vi "VECTOR 1610.vi"() -> ()   [LabVIEW 2020]
uses:
  SubVIs/VECTOR 1610_TypeDefinitions.llb/VECTOR 1610_XL_HWTYPE.ctl
  SubVIs/VECTOR 1610_TypeDefinitions.llb/VECTOR 1610_BitRate.ctl
  SubVIs/VECTOR 1610_TypeDefinitions.llb/VECTOR 1610_Rx_Data.ctl
  LabVIEW 2020 Toolkits/toolkits_lv2020_32bit/Synchronization.llb/SynchRefs_SetGet.ctl
  LabVIEW 2020 Toolkits/VI Server Toolkit/VI Server Libraries/VI Server_GetControl.llb/VI Server_STR_Get.vi
  LabVIEW 2020 Toolkits/VI Server Toolkit/VI Server Libraries/VI Server_Set Controls.llb/Set STR Control.vi
  LabVIEW 2020 Toolkits/VI Server Toolkit/VI Server Libraries/VI Server_GetControl.llb/VI Server_1D_Array_U8_Get.vi
  LabVIEW 2020 Toolkits/VI Server Toolkit/VI Server Libraries/VI Server_SetControl.llb/VI Server_U8_Set.vi
  LabVIEW 2020 Toolkits/VI Server Toolkit/VI Server Libraries/VI Server_GetControl.llb/VI Server_1D_Array_DBL_Get.vi
  LabVIEW 2020 Toolkits/VI Server Toolkit/VI Server Libraries/VI Server_GetControl.llb/VI Server_I32_Get.vi
  LabVIEW 2020 Toolkits/VI Server Toolkit/VI Server Libraries/VI Server_SetControl.llb/VI Server_DBL_Set.vi
  LabVIEW 2020 Toolkits/VI Server Toolkit/VI Server Toolkit LV2013.lvlib
panel:
  in  "LastAction.AddToSecuence":bool
  in  "Open.NIXNET.Database":bool
  in  "Manual.Open":bool caption="IDD.Open"
  in  "IDD.Open":bool
  in  "Help":bool
  in  "FP.Hide":bool caption="FrontPanel.Hide"
  out "System.Message":string caption="System Message"
  in  "EXIT":bool
  in  "Tab.Main":T1(tab)
  in  "TX.Payload.UpdateBytes":bool
  in  "Ch1.TX.Payload.Clear":bool
  in  "CH1.TX.Frames.Cluster":u16(ring) caption="Frames Cluster" items=["NIXNET_Development.CAN_Cluster", "NIXNET_Development.CAN_Demo_Box_Cluster", "NIXNET_Development.FlexRay_Cluster", "NIXNET_Development.J1939_Over_CAN"]
  out "CH1.TX.Signal.Comment":string caption="Comment"
  out "CH1.TX.Frame.PayloadLength":u32 caption="Payload Length"
  out "CH1.TX.Frame.Identifier":u32 caption="Identifier" format="%08x"
  in  "CH1.TX.Frame.Selector":u16(ring) caption="Frame Selector"
  out "CH1.TX.Signal.Unit":string caption="Unit"
  out "CH1.TX.Signal.DefaultValue":dbl caption="Default Value"
  out "CH1.TX.Signal.MinimumValue":dbl caption="Minimum Value"
  out "CH1.TX.Signal.MaximumValue":dbl caption="Maximum Value"
  out "CH1.TX.Signal.ScalingOffset":dbl caption="Scaling Offset"
  out "CH1.TX.Signal.ScalingFactor":dbl caption="Scaling Factor"
  out "CH1.TX.Signal.ByteOrder":u32(ring) caption="Byte Order" items=["Little Endian", "Big Endian"]
  out "CH1.TX.Signal.DataType":u32(ring) caption="Data Type" items=["Signed", "Unsigned", "IEEE Float"]
  out "CH1.TX.Signal.NumberOfBits":u32 caption="Number Of Bits"
  out "CH1.TX.Signal.StartBit":u32 caption="Start Bit"
  out "CH1.TX.Signal.Name":string caption="Name"
  in  "CH1.TX.Frame.Signals":u16(ring) caption="Frame Signals"
  in  "Ch1.TX.Transmit.Byte8":u8 caption="Byte 8" format="%02x"
  in  "Ch1.TX.Transmit.Byte7":u8 caption="Byte 7" format="%02x"
  in  "Ch1.TX.Transmit.Byte6":u8 caption="Byte 6" format="%02x"
  in  "Ch1.TX.Transmit.Byte5":u8 caption="Byte 5" format="%02x"
  in  "Ch1.TX.Transmit.Byte4":u8 caption="Byte 4" format="%02x"
  in  "Ch1.TX.Transmit.Byte3":u8 caption="Byte 3" format="%02x"
  in  "Ch1.TX.Transmit.Byte2":u8 caption="Byte 2" format="%02x"
  in  "Ch1.TX.Transmit.Byte1":u8 caption="Byte 1" format="%02x"
  in  "Ch1.TX.DataLength":u16 caption="Data Length" max=8
  in  "CH1.TX.FrameID":u32=2566838656 caption="Frame ID" format="%08x"
  in  "Ch1.TX.Payload":u8[](array[numeric]) caption="Payload" format="%02x"
  in  "CH1.TX.Signal.Data":dbl caption="Signal Data" min=0.0 max=10000.0 format="%0.3f "
  in  "Ch1.TX.Transmit":bool
  out "Ch2.ReceivedDataArray.IndexedValue":dbl caption="Value" format="%0.0f"
  in  "Ch2.ReceivedDataArray.Index":i32 caption="Index" max=6
  in  "Ch2.ReceivedDataArray.Precision":u8 caption="Precision" max=6
  out "Ch2.ReceivedDataArray":dbl[](array[numeric]) caption="Received Data Array"
  out "Ch2.Responce.String":string
  out "Ch1.Responce.Message.Checksum":string caption="Checksum"
  out "Ch1.Responce.Message.Load":string caption="PayloadLoad"
  out "Ch1.Responce.Message.Length":string caption="Length"
  out "Ch1.Responce.Message.ID":string caption="Message ID"
  out "Ch1.Responce.Message.Payload":u8[](array[numeric]) caption="Message Payload" format="%02x"
  out "CH1.RX.Signal.Data":dbl caption="Signal Data" min=0.0 max=8031.000000000005 format="%0.3f rpm"
  out "CH1.RX.Signal.Unit":string caption="Unit"
  out "CH1.RX.Signal.DefaultValue":dbl caption="Default Value"
  out "CH1.RX.Signal.MinimumValue":dbl caption="Minimum Value"
  out "CH1.RX.Signal.MaximumValue":dbl caption="Maximum Value"
  out "CH1.RX.Signal.ScalingOffset":dbl caption="Scaling Offset"
  out "CH1.RX.Signal.ScalingFactor":dbl caption="Scaling Factor"
  out "CH1.RX.Signal.ByteOrder":u32(ring) caption="Byte Order" items=["Little Endian", "Big Endian"]
  out "CH1.RX.Signal.DataType":u32(ring) caption="Data Type" items=["Signed", "Unsigned", "IEEE Float"]
  out "CH1.RX.Signal.NumberOfBits":u32 caption="Number Of Bits"
  out "CH1.RX.Signal.StartBit":u32 caption="Start Bit"
  in  "CH1.RX.FrameIDs":u16(ring) caption="Frame Id's"
  out "CH1.RX.Frame.PayloadLength":u32 caption="Payload Length"
  out "CH1.RX.Frame.Identifier":u32 caption="Identifier" format="%.0x"
  in  "CH1.RX.Frame.Selector":u16(ring) caption="Frame Selector"
  out "CH1.RX.Signal.Name":string caption="Name"
  in  "CH1.RX.Frame.Signals":u16(ring) caption="Frame Signals"
  out "CH1.RX.DATA":T2[](array[typedef]) caption="RX DATA" {"TimeStamp" format="%.0x"; "CH1.Received.Payload" format="%02x"; "CH1.Received.DataLength" max=8; "CH1.Received.FrameID" format="%08x"}
  out "CH1.RX.Signal.Comment":string caption="Comment"
  in  "CH1.RX.Frames.Cluster":u16(ring) caption="Frames Cluster" items=["NIXNET_Development.CAN_Cluster", "NIXNET_Development.CAN_Demo_Box_Cluster", "NIXNET_Development.FlexRay_Cluster", "NIXNET_Development.J1939_Over_CAN"]
  out "StringMode.Received Data":string
  in  "Argument.Precision":u8 caption="Precision" max=6
  in  "Argument.Value":dbl caption="Value"
  in  "Argument.Number":i32=1 caption="Number" min=1 max=100
  in  "Message.PrototypeString":string caption="Message Prototype String"
  in  "TestCase.Execute.All":bool
  in  "TestCase.Execute.Selected":bool
  out "TestCase.SAVE.Success":bool
  in  "TestCase.SAVE":bool
  in  "SequenceFile.Open":bool
  in  "SequenceFile":path caption="Secuence File"
  in  "TestCase.Execute.Step.Pause":bool
  in  "TestCase.Execute.Steps":u16(ring) caption="Test Case: Pause Before Step" items=["1", "2", "3", "4", "5", "6", "7", "8", "9", "10", "11", "12", "13", "14", "15", "16", "17", "18"]
  in  "TestCase.Execute.ABORT":bool
  in  "TestCase.Execute.Next":bool
  in  "TestCase.Execute.Pause":bool
  out "TestCase.ExecutionTime":dbl caption="Execution Time:" format="%0.3f sec"
  in  "TestCase.Execution.StepTime":u32 caption="Seq. Execution: Step Time" format="%d msec"
  in  "TestCaseConfiguration":i32[](listbox) caption="Test Case Configuration"
  in  "TestCase.StepDescription":string caption="Step Description:"
  in  "NIXNET.DatabaseEditor":path=path "C:/Program Files (x86)/National Instruments/NI-XNET/editor/XNetDbEd.exe" caption="NIXNET Database Editor"
  in  "Database.Selector":u16(ring) caption="Database Selector" items=["NIXNET_Development", "NIXNET_Development_1", "NIXNET_Development_2", "NIXNET_Development_3"]
  in  "BitRate":T3=125000 caption="Bit Rate" items=["20 KBd"=20000, "50 KBd"=50000, "62K5 Bd"=62500, "100 KBd"=100000, "125 KBd"=125000, "250 KBd"=250000, "500 KBd"=500000, "1 MBd"=1000000]
  in  "hwChannel.1":i32
  in  "hwIndex":i32
  in  "XL_HWTYPE":T4=55 items=["NONE"=0, "VIRTUAL"=1, "CANCARDX"=2, "CANCARDY"=12, "CANCARDXL"=15, "CANCASEXL"=21, "CANCASEXL_LOG_OBSOLETE"=23, "CANBOARDXL"=25, "CANBOARDXL_PXI"=27, "VN2600"=29, "VN3300"=37, "VN3600"=39, "VN7600"=41, "CANCARDXLE"=43, "VN8900"=45, "VN8950"=47, "VN2640"=53, "VN1610"=55, "VN1630"=57, "VN1640"=59, "VN8970"=61, "VN1611"=63, "VN5610"=65, "VN7570"=67, "IPCLIENT"=69]
  in  "VI.WindowsTitle":string caption="Windows Title"
  in  "UDP.Test.String2.Send":bool
  in  "UDP.Test.String2":string caption="UDP: Test String 2"
  in  "UDP.Port.BC":u16=58433 caption="UDP: Port.BC"
  in  "UDP.Port.RT":u16=58432 caption="UDP: Port.RT"
  in  "UDP.LocalPort.Write":u16=58434 caption="UDP: Local Port.Write"
  in  "UDP.IP.Address":string="234.5.6.7" caption="UDP: IP Address"
  in  "UDP.Test.String1.Send":bool
  in  "UDP.Test.String1":string caption="UDP: Test String 1"
  in  "UDP.Responce.String.Monitor":bool
  out "UDP.ExecEng.Message.String":string caption="UDP: Execution Engine Message String"
  out "error out":errorcluster
  in  "hwChannel.2":i32
  in  "error in":errorcluster
  # "13JUN2022"
  # "Channel 1 Send Data"
  # "Channel 1 Received Data"
  # "M"
  # "VESTOR 1610 SETTINGS"
  # "Multicast IP addresses must be in the 224.0.0.0 to 239.255.255.255 range."
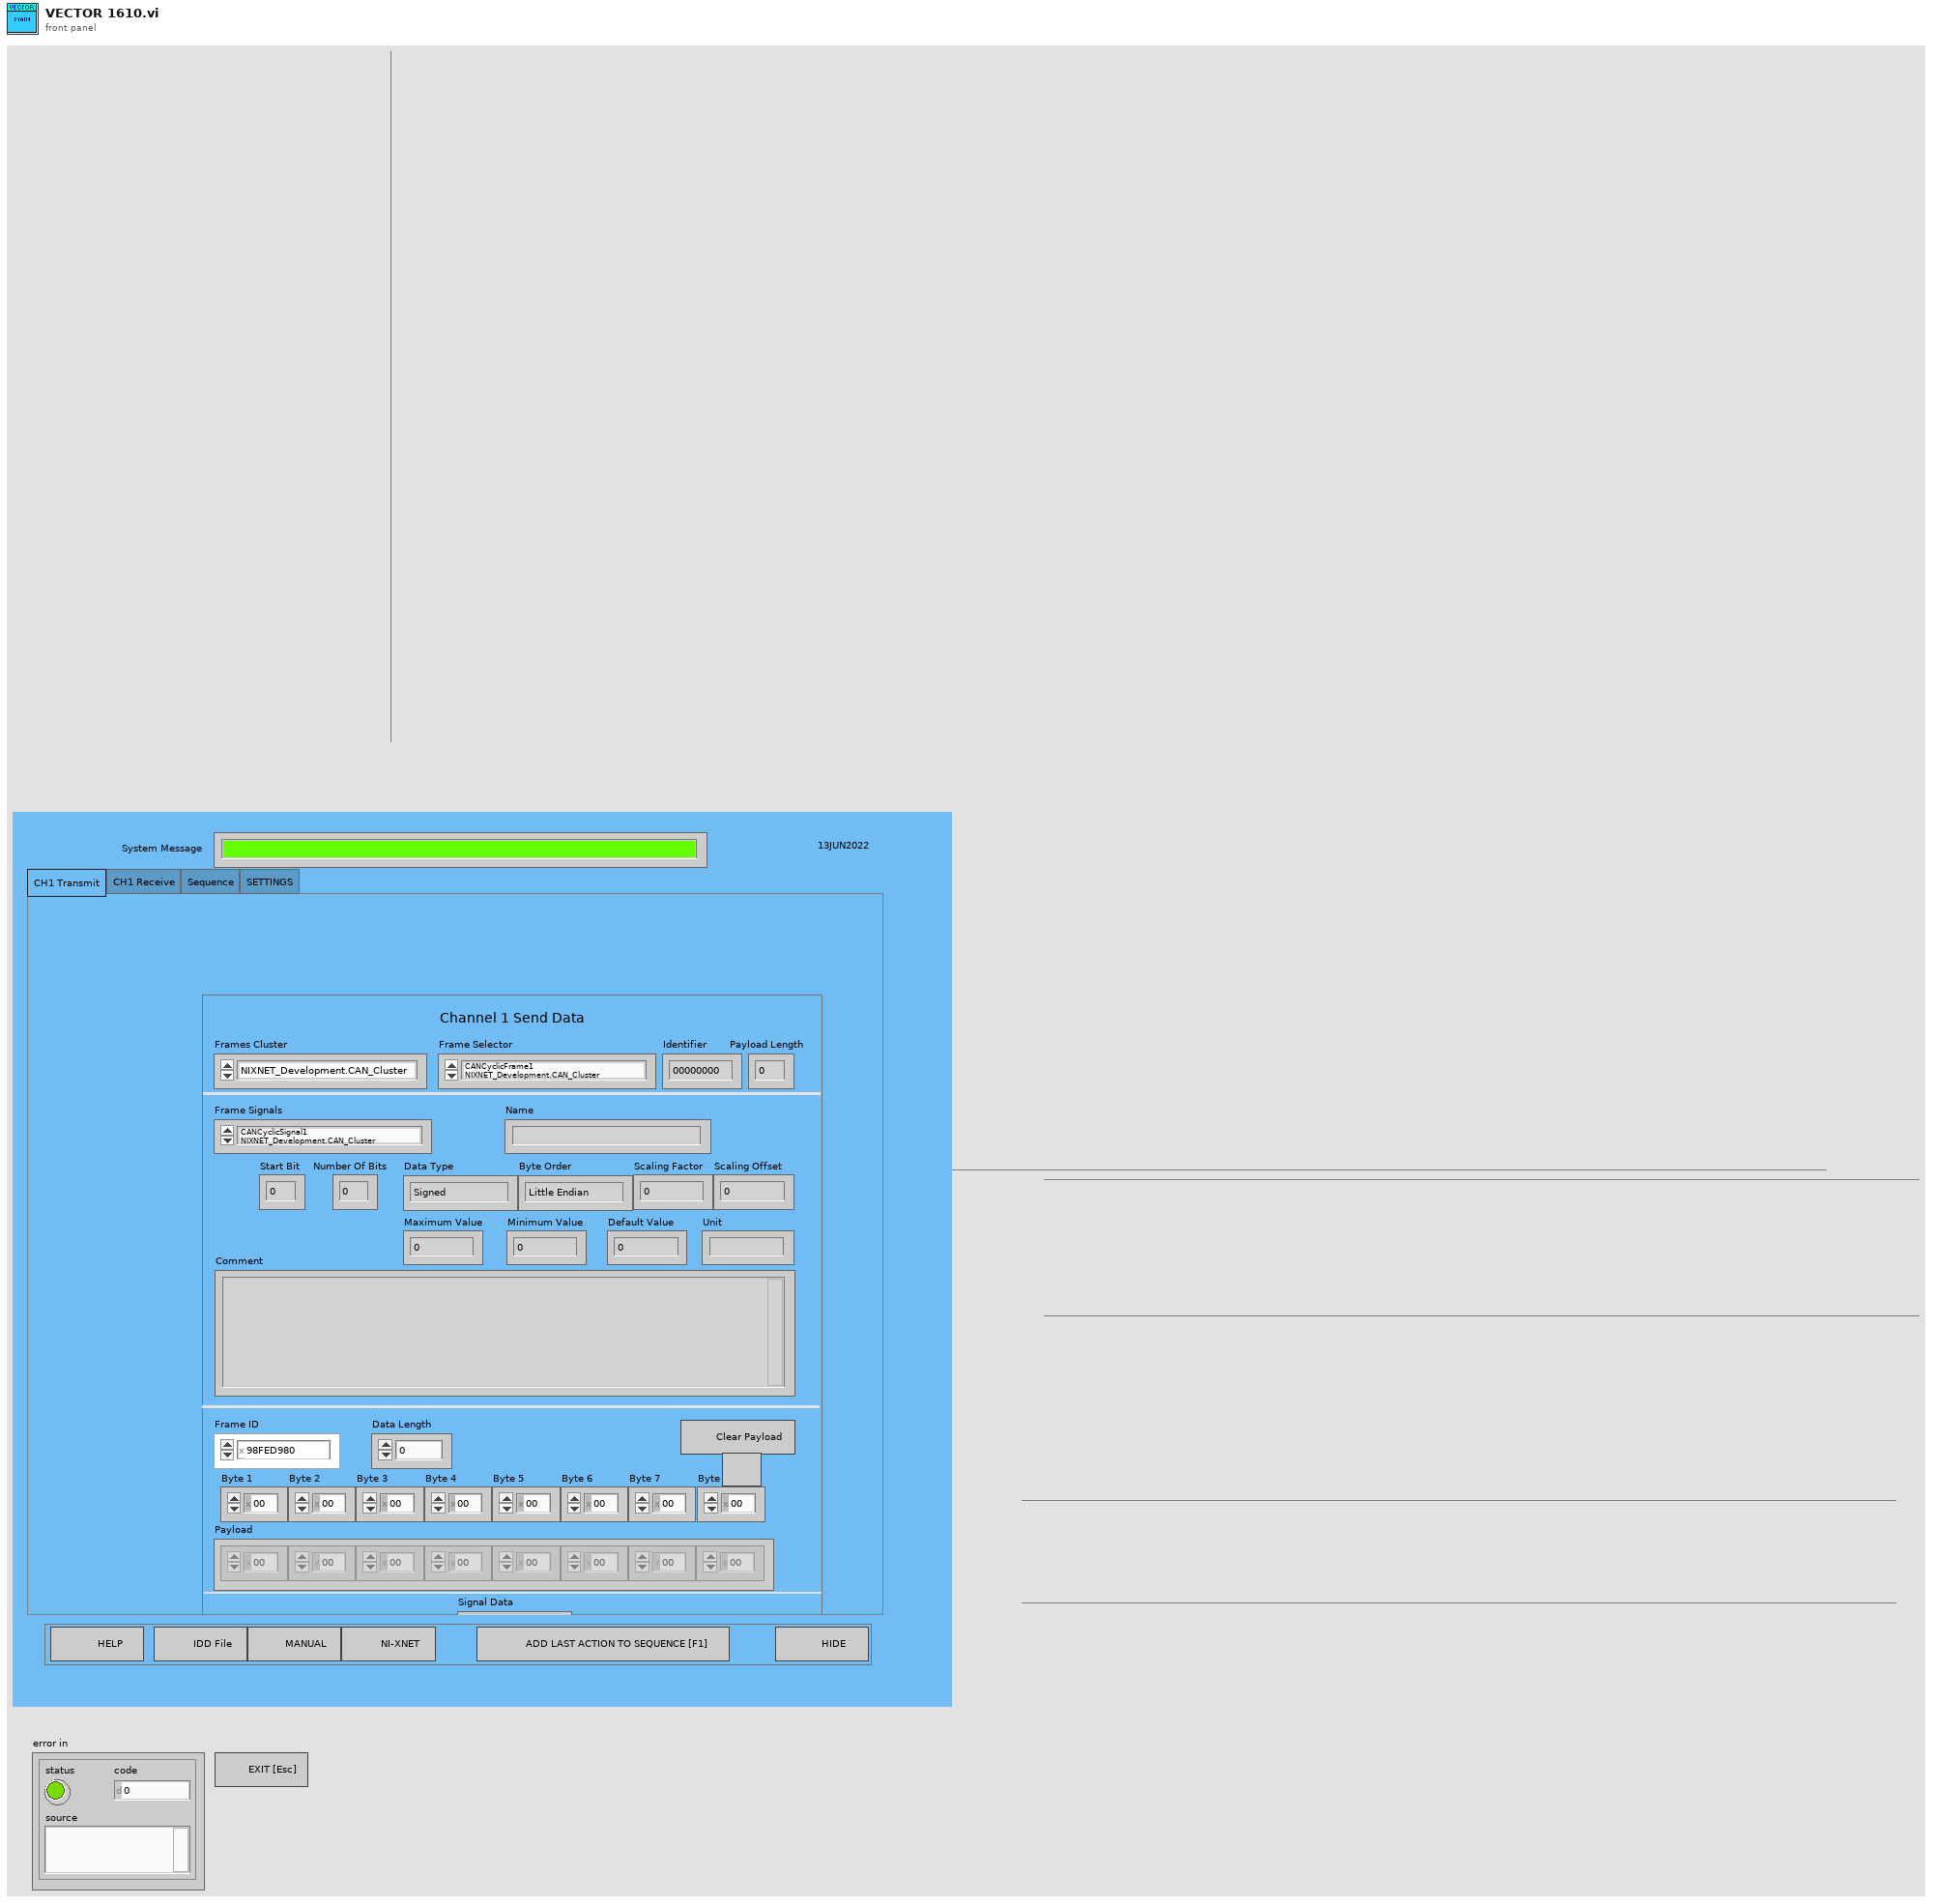
[diagram p1: front panel]
types:
  T1 = enum32{"CH1 Transmit", "CH1 Receive", "Sequence", "SETTINGS"}
  T2 = typedef "VECTOR 1610_Rx_Data.ctl" = cluster{"CH1.Received.Payload":u8[], "CH1.Received.DataLength":u16, "CH1.Received.FrameID":u32, "TimeStamp":u64}
  T3 = typedef "VECTOR 1610_BitRate.ctl" = u32
  T4 = typedef "VECTOR 1610_XL_HWTYPE.ctl" = u8
  T5 = typedef "VI Server_RefsCluster.ctl" = cluster{"Labels":string[], "Refs":refnum<vi>[], "VI Ref":refnum<vi>}
  T6 = typedef "SynchRefs_SetGet.ctl" = enum16{"Set", "Get"}
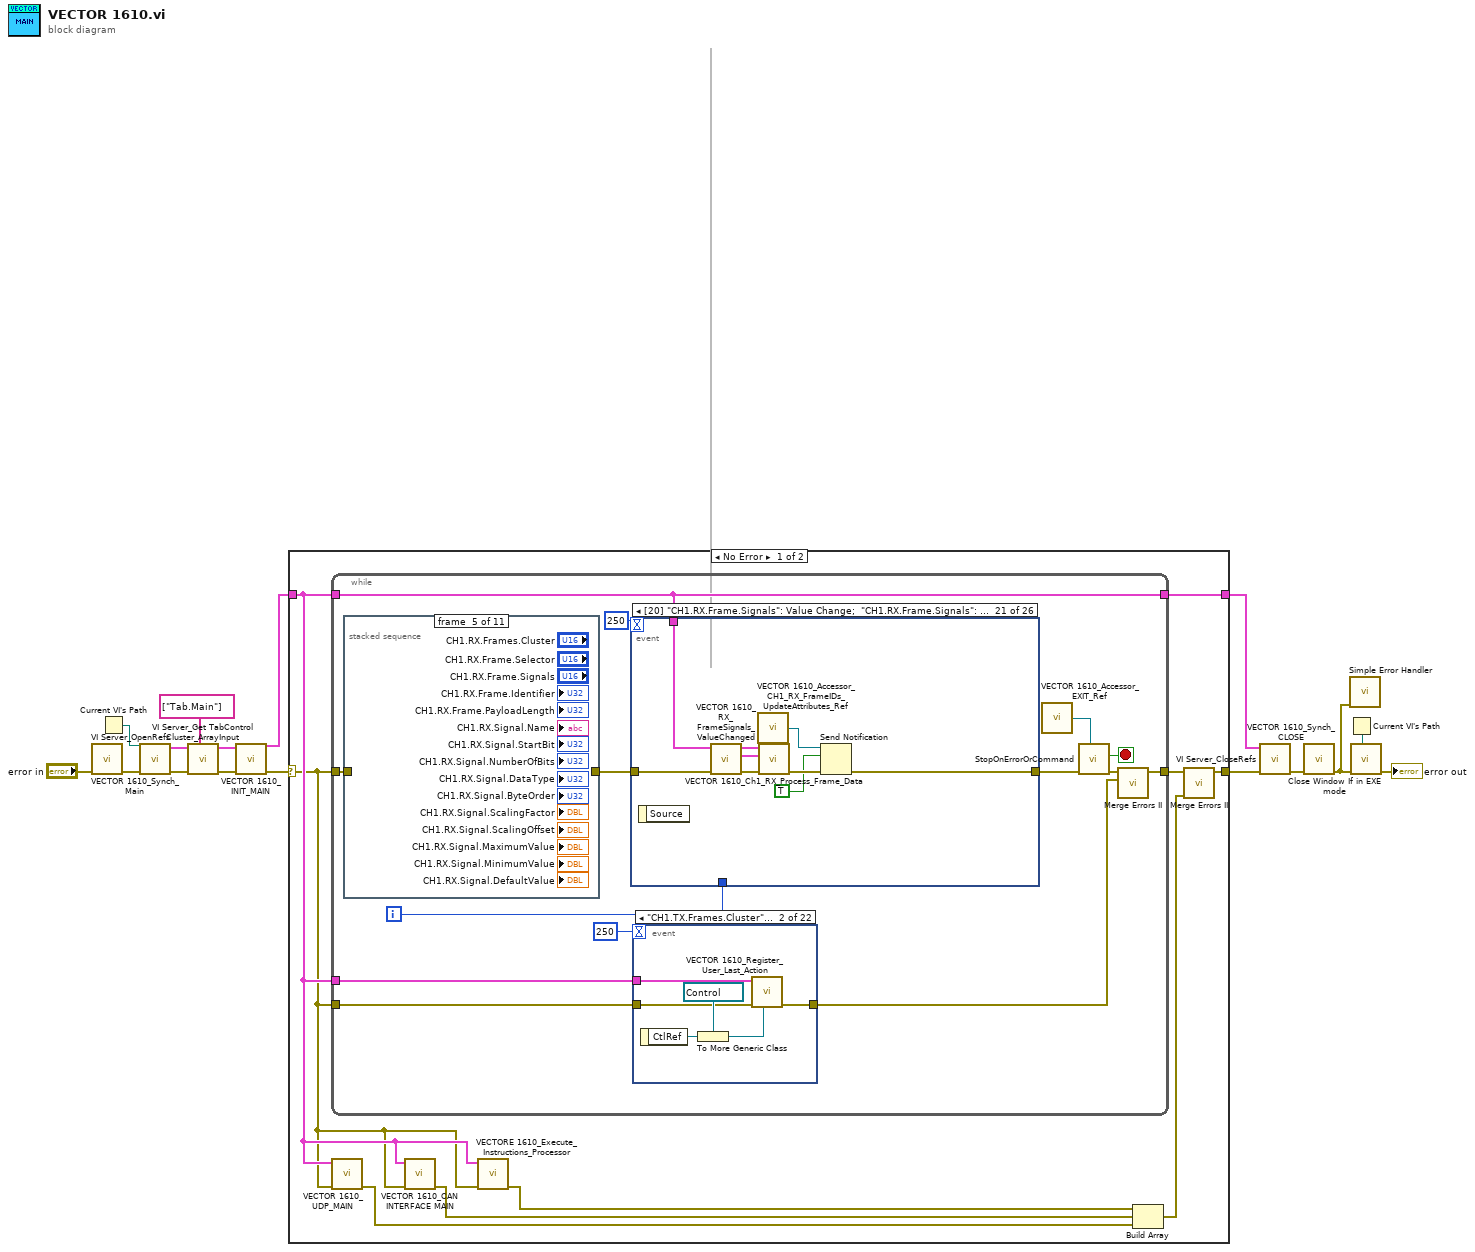
[diagram p0: block diagram]
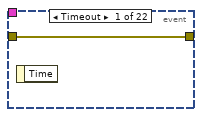
[diagram p2: hidden frame]
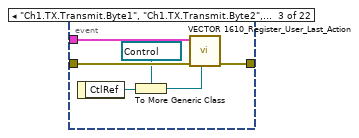
[diagram p3: hidden frame]
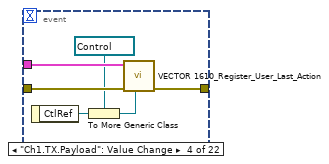
[diagram p4: hidden frame]
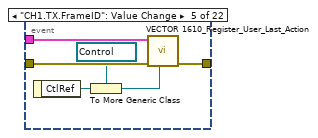
[diagram p5: hidden frame]
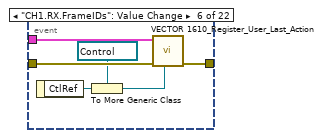
[diagram p6: hidden frame]
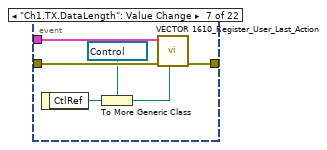
[diagram p7: hidden frame]
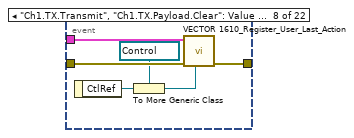
[diagram p8: hidden frame]
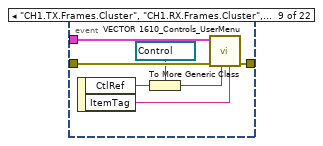
[diagram p9: hidden frame]
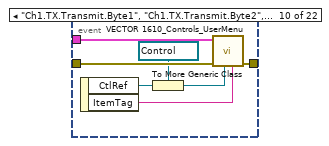
[diagram p10: hidden frame]
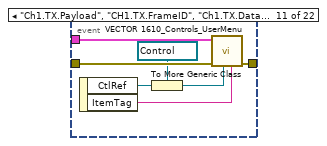
[diagram p11: hidden frame]
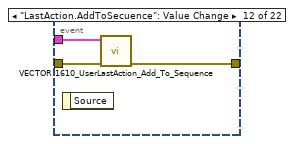
[diagram p12: hidden frame]
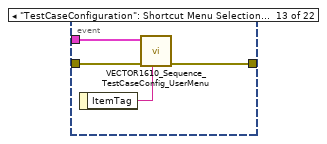
[diagram p13: hidden frame]
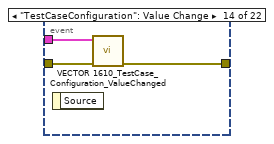
[diagram p14: hidden frame]
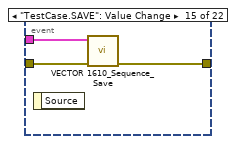
[diagram p15: hidden frame]
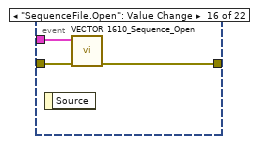
[diagram p16: hidden frame]
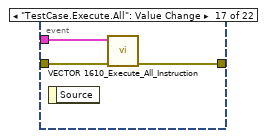
[diagram p17: hidden frame]
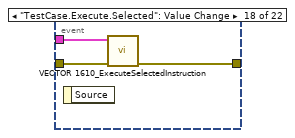
[diagram p18: hidden frame]
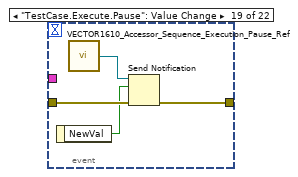
[diagram p19: hidden frame]
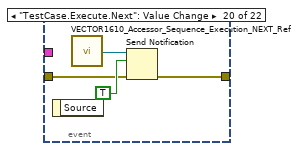
[diagram p20: hidden frame]
diagram:
  n1 = call "VECTOR 1610_Synch_Main.vi"("error in"="error in") -> ("error out"=w11:errorcluster)  [unwired: 10 in]
  n2 = Current VI's Path() -> (path=w15:path)
  n3 = call "VI Server_OpenRefs.vi"("error in"=w11, "VI Path"=w15) -> ("error out"=w12:errorcluster, "VI Server.RefsCluster"=w13:T5)  [unwired: 8 in]
  n4 = call "VI Server_Get TabControl Cluster_ArrayInput.vi"("TabControl Labels[]"=string[] ["Tab.Main"], "error in"=w12, "VI Server Cluster"=w13) -> ("error out"=w10:errorcluster, "VI Server Cluster.OUT"=w9:T5)  [unwired: 7 in]
  n5 = call "VECTOR 1610_INIT_MAIN.vi"("error in (no error)"=w10, "VI Server Cluster"=w9) -> ("error out"=w8:errorcluster, "VI Server Cluster DUP"=w1:T5)  [unwired: 8 in]
  n6 = case shown="No Error" w8 {
    selector: w8 -> [w18 w304]
    tunnel: [w22 w304] -> w3
    tunnel: w1 -> [w19 w303]
    tunnel: [w25 w303] -> w4
    frame No Error {
      n7 = while {
        tunnel: w18 -> [w39]
        tunnel: [w27] -> w23
        tunnel: w19 -> [w35]
        tunnel: [w35] -> w25
        tunnel: w19 -> [w30]
        tunnel: w18 -> [w29]
        i -> [w36]
        stop <- w33 stop-if-true
        n8 = stacked-sequence {
          tunnel: w39 -> [w302 _ _ _ _ _ _ _ _ _ _]
          tunnel: [w302 _ _ _ _ _ _ _ _ _ _] -> w38
          frame #0 {
          }
          frame #1 {
          }
          frame #2 {
          }
          frame #3 {
          }
          frame #4 {
          }
          frame #5 {
          }
          frame #6 {
          }
          frame #7 {
          }
          frame #8 {
          }
          frame #9 {
          }
          frame #10 {
          }
        }
        n9 = event shown="[20] \"CH1.RX.Frame.Signals\": Value Change;  \"CH1.RX.Frame.Signals\": Mouse Up" {
          selector: _ -> [_ _ _ _ _ _ _ _ _ _ _ _ _ _ _ _ _ _ _ _ _ _ _ _ _ _]
          dyn-events: _ -> [_ _ _ _ _ _ _ _ _ _ _ _ _ _ _ _ _ _ _ _ _ _ _ _ _ _]
          timeout: 250 -> [_ _ _ _ _ _ _ _ _ _ _ _ _ _ _ _ _ _ _ _ _ _ _ _ _ _]
          tunnel: w38 -> [w145 w147 w156 w159 w163 w172 w181 w185 w205 w214 w217 w222 w225 w228 w238 w251 w254 w255 w260 w263 w272 w275 w278 w282 w285 w301]
          tunnel: w36 -> [w144 _ _ _ _ _ _ _ _ _ _ _ _ _ _ _ _ _ _ _ _ _ _ _ _ _]
          tunnel: [w142 w149 w157 w159 w161 w170 w179 w183 w206 w215 w218 w219 w224 w226 w231 w250 w252 w256 w259 w261 w266 w273 w276 w280 w284 w286] -> w34
          tunnel: w35 -> [w143 _ w153 _ _ w169 w178 w182 w204 w213 w216 _ w223 w227 w237 w249 w253 w257 w258 w262 w271 w274 w277 w281 w283 w300]
          event Timeout {
            n10 = event-data() -> ()  [unwired: 1 in, 1 out]
            n11 = call "VECTOR 1610_UserLastSelection_Set_Get.vi"("LoopCounter"=w144, "SynchRefs.Set/Get"=SynchRefs_SetGet."Set", "error in"=w145, "VI Server.RefsCluster"=w143) -> ("error out"=w142:errorcluster)  [unwired: 6 in, 1 out]
          }
          event "EXIT": Value Change {
            n12 = event-data() -> ()  [unwired: 1 in, 1 out]
            n13 = call "VECTOR 1610_Accessor_EXIT_Ref.vi"() -> ("EXIT"=w150:refnum<notifier>)  [unwired: 6 in]
            n14 = Send Notification(notification=TRUE, notifier=w150, error in (no error)=w147) -> (error out=w149:errorcluster)  [unwired: 1 out]
          }
          event "FP.Hide": Value Change {
            n15 = event-data() -> ("NewVal"=w154:bool)  [unwired: 1 in]
            n16 = call "VECTOR 1610_Accessor_FP_State_Ref.vi"() -> ("FP.State"=w151:refnum<notifier>)  [unwired: 6 in]
            n17 = call "ExecEng_InstrumentsFrontPanel_Hide_Show.vi"("FP.Hide/Show"=w154, "FP.State"=w151, "error in (no error)"=w156, "VI Server Cluster"=w153) -> ("error out"=w155:errorcluster, "VI Server Cluster DUP"=w152:T5)  [unwired: 6 in]
            n18 = call "VECTOR 1610_FP_Hide_SendMessageToExecEng.vi"("error in (no error)"=w155, "VI Server Cluster"=w152) -> ("error out"=w157:errorcluster)  [unwired: 9 in]
          }
          event "Help": Value Change {
            n19 = event-data() -> ("NewVal"=w158:bool)  [unwired: 1 in]
            n20 = Control Help Window(1:w158) -> ()  [unwired: 1 in]
          }
          event "UDP.Responce.String.Monitor": Value Change {
            n21 = event-data() -> ("NewVal"=w160:bool)  [unwired: 1 in]
            n22 = call "VECTOR 1610_Accessor_UDP_Responce_String_Monitor_Ref.vi"() -> ("UDP.ExecEng.Command.String.Monitor"=w162:refnum<notifier>)  [unwired: 6 in]
            n23 = Send Notification(notification=w160, notifier=w162, error in (no error)=w163) -> (error out=w161:errorcluster)  [unwired: 1 out]
          }
          event "UDP.Test.String1.Send": Value Change {
            n24 = event-data() -> ()  [unwired: 1 in, 1 out]
            n25 = call-poly "VI Server_GetControl_Value_Ref.vi"("DataType"="", "Control.Label"="UDP.Test.String1", "error in"=w172, "SingleInstance"=TRUE, "VI Server.RefsCluster"=w169) -> ("error out"=w171:errorcluster, "Value"=w164:string)  [unwired: 3 in, 2 out]
            n26 = call "VECTOR 1610_Accessor_UDP_Instrument_Responce_Ref.vi"() -> ("UDP.Instrument.Responce.Q"=w165:refnum<queue>)  [unwired: 6 in]
            n27 = Enqueue Element(queue=w165, element=w164, error in (no error)=w171) -> (error out=w170:errorcluster)  [unwired: 1 in, 2 out]
          }
          event "UDP.Test.String2.Send": Value Change {
            n28 = event-data() -> ()  [unwired: 1 in, 1 out]
            n29 = call-poly "VI Server_GetControl_Value_Ref.vi"("DataType"="", "Control.Label"="UDP.Test.String2", "error in"=w181, "SingleInstance"=TRUE, "VI Server.RefsCluster"=w178) -> ("error out"=w180:errorcluster, "Value"=w173:string)  [unwired: 3 in, 2 out]
            n30 = call "VECTOR 1610_Accessor_UDP_Instrument_Responce_Ref.vi"() -> ("UDP.Instrument.Responce.Q"=w174:refnum<queue>)  [unwired: 6 in]
            n31 = Enqueue Element(queue=w174, element=w173, error in (no error)=w180) -> (error out=w179:errorcluster)  [unwired: 1 in, 2 out]
          }
          event "UDP.ExecEng.Message.String": Shortcut Menu Selection (User) {
            n32 = event-data() -> ("ItemTag"=w184:string)  [unwired: 1 in]
            n33 = case shown="\"Clear Indicator\"" w184 {
              tunnel: w185 -> [w186 w192]
              tunnel: [w186 w191] -> w183
              tunnel: w182 -> [_ w190]
              frame "", Default {
              }
              frame "Clear Indicator" {
                n34 = call-poly "VI Server_Set Control Value.vi"("New Value"="", "Label"="UDP.ExecEng.Message.String" ("Control.Label"), "error in"=w192, "Single Instance (T)"=TRUE ("SingleInstance"), "VI Server Cluster"=w190) -> ("error out"=w191:errorcluster)  [unwired: 4 in, 2 out]
              }
            }
          }
          event "IDD.Open": Value Change {
            n35 = event-data() -> ()  [unwired: 1 in, 1 out]
            n36 = call "VI Server_Get Text Ring Selection.vi"("Label"="Protocol", "error in"=w205, "Single Instance (T)"=TRUE, "VI Server Cluster"=w204) -> ("error out"=w194:errorcluster, "Selection"=w201:string)  [unwired: 2 in, 4 out]
            n37 = call "VECTOR 1610_GetProtocolPath.vi"("VI Server Cluster"=w204, "Protocol.Name"=w201) -> ("Protocol.Path"=w200:path)  [unwired: 3 in, 2 out]
            n38 = Path To String(path=w200) -> (string=w199:string)
            n39 = Search and Replace String(input string=w199, search string=".cfg", replace string=".pdf" ("replace string (\"\")"), error in=w194) -> (result string=w196:string, error out=w193:errorcluster)  [unwired: 4 in, 2 out]
            n40 = String To Path(string=w196) -> (path=w195:path)
            n41 = call "ExecEng_Instrument_OpenOperatorManual.vi"("Operations Manual Path"=w195, "error in"=w193, "VI Server.RefsCluster"=w204) -> ("error out"=w206:errorcluster)  [unwired: 8 in]
          }
          event "Manual.Open": Value Change {
            n42 = event-data() -> ()  [unwired: 1 in, 1 out]
            n43 = call "VI Server_GenerateConfigurationFolderPath_ClusterInput.vi"("VI Server Cluster"=w213) -> ("Configuration Folder Path"=w212:path)  [unwired: 11 in, 3 out]
            n44 = Strip Path(path=w212) -> (stripped path=w211:path)  [unwired: 1 out]
            n45 = Build Path(base path=w211, name or relative path="DOCs") -> (appended path=w209:path)
            n46 = Build Path(base path=w209, name or relative path="Soft Panel Manual.pdf") -> (appended path=w207:path)
            n47 = call "ExecEng_Instrument_OpenOperatorManual.vi"("Operations Manual Path"=w207, "error in"=w214, "VI Server.RefsCluster"=w213) -> ("error out"=w215:errorcluster)  [unwired: 8 in]
          }
          event "Open.NIXNET.Database": Value Change {
            n48 = event-data() -> ()  [unwired: 1 in, 1 out]
            n49 = call "VECTOR 1610_OpenNIXNETl.vi"("error in"=w217, "VI Server.RefsCluster"=w216) -> ("error out"=w218:errorcluster)  [unwired: 9 in]
          }
          event "hwIndex", "hwChannel.1", "hwChannel.2": Value Change {
            n50 = event-data() -> ()  [unwired: 1 in, 1 out]
            n51 = call "VECTOR 1610_Accessor_RST_Ref.vi"() -> ("RST"=w221:refnum<notifier>)  [unwired: 6 in]
            n52 = Send Notification(notification=TRUE, notifier=w221, error in (no error)=w222) -> (error out=w219:errorcluster)  [unwired: 1 out]
          }
          event "Database.Selector": Value Change {
            n53 = event-data() -> ()  [unwired: 1 in, 1 out]
            n54 = call "VECTOR 1610_PopulateFrameCluster.vi"("error in (no error)"=w225, "VI Server Cluster"=w223) -> ("error out"=w224:errorcluster)  [unwired: 8 in, 1 out]
          }
          event "Ch1.TX.Payload.Clear": Value Change {
            n55 = event-data() -> ()  [unwired: 1 in, 1 out]
            n56 = call "VECTOR 1610_TX_Payload_Clear.vi"("error in (no error)"=w228, "VI Server Cluster"=w227) -> ("error out"=w226:errorcluster)  [unwired: 9 in]
          }
          event "TX.Payload.UpdateBytes": Value Change {
            n57 = event-data() -> ()  [unwired: 1 in, 1 out]
            n58 = call-poly "VI Server_GetControl_Value_Ref.vi"("DataType"=u8[] [] ("Ch1.TX.Payload 2"), "Control.Label"="Ch1.TX.Payload", "error in"=w238, "SingleInstance"=TRUE, "VI Server.RefsCluster"=w237) -> ("error out"=w233:errorcluster, "Value"=w230:u8[], "VI Server.RefsCluster.DUP"=w232:T5)  [unwired: 3 in, 1 out]
            n59 = for {
              tunnel: w232 -> [w248]
              tunnel: w233 -> [w243]
              tunnel: [w246] -> w231
              tunnel: w230 -> [w245] mode=indexing
              tunnel: "Ch1.TX.Transmit.Byte%d" -> [w240]
              i -> [w242]
              stop <- w246 stop-if-true
              n60 = Increment(x=w242) -> (x+1=w241:i32)
              n61 = Format Into String(format string=w240, error in=w243, w241) -> (resulting string=w239:string, error out=w244:errorcluster)  [unwired: 1 in]
              n62 = call-poly "VI Server_SetControl.vi"("Data"=w245, "Control.Label"=w239, "error in"=w244, "SingleInstance"=FALSE, "VI Server.RefsCluster"=w248) -> ("error out"=w246:errorcluster)  [unwired: 4 in, 2 out]
            }
          }
          event "CH1.TX.Frames.Cluster": Value Change {
            n63 = event-data() -> ()  [unwired: 1 in, 1 out]
            n64 = call "VECTOR 1610_CH1_TX_FrameCluster_ValueChanged.vi"("error in (no error)"=w251, "VI Server Cluster"=w249) -> ("error out"=w250:errorcluster)  [unwired: 8 in, 1 out]
          }
          event "CH1.RX.Frames.Cluster": Value Change {
            n65 = event-data() -> ()  [unwired: 1 in, 1 out]
            n66 = call "VECTOR 1610_CH1_RX_FrameCluster_ValueChanged.vi"("error in (no error)"=w254, "VI Server Cluster"=w253) -> ("error out"=w252:errorcluster)  [unwired: 8 in, 1 out]
          }
          event "CH1.TX.Frame.Selector": Value Change; "CH1.TX.Frame.Selector": Mouse Up {
            n67 = event-data() -> ()  [unwired: 1 in, 1 out]
            n68 = call "VECTOR 1610_FrameSelector_ValueChanged.vi"("error in (no error)"=w255, "VI Server Cluster"=w257) -> ("error out"=w256:errorcluster)  [unwired: 8 in, 1 out]
          }
          event "CH1.RX.Frame.Selector": Value Change; "CH1.RX.Frame.Selector": Mouse Up {
            n69 = event-data() -> ()  [unwired: 1 in, 1 out]
            n70 = call "VECTOR 1610_RX_FrameSelector_ValueChanged.vi"("error in (no error)"=w260, "VI Server Cluster"=w258) -> ("error out"=w259:errorcluster)  [unwired: 8 in, 1 out]
          }
          event "CH1.TX.Frame.Signals": Value Change; "CH1.TX.Frame.Signals": Mouse Up {
            n71 = event-data() -> ()  [unwired: 1 in, 1 out]
            n72 = call "VECTOR 1610_FrameSignals_ValueChanged.vi"("error in (no error)"=w263, "VI Server Cluster"=w262) -> ("error out"=w261:errorcluster)  [unwired: 8 in, 1 out]
          }
          event "CH1.RX.Frame.Signals": Value Change; "CH1.RX.Frame.Signals": Mouse Up {
            n73 = event-data() -> ()  [unwired: 1 in, 1 out]
            n74 = call "VECTOR 1610_RX_FrameSignals_ValueChanged.vi"("error in (no error)"=w272, "VI Server Cluster"=w271) -> ("error out"=w270:errorcluster, "Rx.DATA"=w268:T2, "VI Server Cluster DUP"=w269:T5)  [unwired: 7 in]
            n75 = call "VECTOR 1610_Accessor_CH1_RX_FrameIDs_UpdateAttributes_Ref.vi"() -> ("CH1.RX.FrameIDs.UpdateAttributes"=w265:refnum<notifier>)  [unwired: 6 in]
            n76 = call "VECTOR 1610_Ch1_RX_Process_Frame_Data.vi"("error in (no error)"=w270, "Rx.DATA"=w268, "VI Server Cluster"=w269) -> ("error out"=w267:errorcluster)  [unwired: 8 in]
            n77 = Send Notification(notification=TRUE, notifier=w265, error in (no error)=w267) -> (error out=w266:errorcluster)  [unwired: 1 out]
          }
          event "CH1.RX.FrameIDs": Value Change; "CH1.RX.FrameIDs": Mouse Up {
            n78 = event-data() -> ()  [unwired: 1 in, 1 out]
            n79 = call "VECTOR 1610_Ch1_RX_FrameID_Changed.vi"("error in (no error)"=w275, "VI Server Cluster"=w274) -> ("error out"=w273:errorcluster)  [unwired: 9 in]
          }
          event "CH1.TX.Signal.Data": Value Change {
            n80 = event-data() -> ()  [unwired: 1 in, 1 out]
            n81 = call "VECTOR 1610_Ch1_SignalData_ValueChanged.vi"("error in (no error)"=w278, "VI Server Cluster"=w277) -> ("error out"=w276:errorcluster)  [unwired: 8 in, 1 out]
          }
          event "Ch1.TX.Transmit.Byte1", "Ch1.TX.Transmit.Byte2", "Ch1.TX.Transmit.Byte3", "Ch1.TX.Transmit.Byte4", "Ch1.TX.Transmit.Byte5", "Ch1.TX.Transmit.Byte6", "Ch1.TX.Transmit.Byte7", "Ch1.TX.Transmit.Byte8": Value Change {
            n82 = event-data() -> ("CtlRef"=w279:refnum<vi>)  [unwired: 1 in]
            n83 = call "VECTOR 1610_Finctions_Ch1_FormatData.vi"("CtlRef"=w279, "error in (no error)"=w282, "VI Server Cluster"=w281) -> ("error out"=w280:errorcluster)  [unwired: 8 in]
          }
          event "Ch1.TX.Transmit": Value Change {
            n84 = event-data() -> ()  [unwired: 1 in, 1 out]
            n85 = call "VECTOR 1610_Ch1_Transmit.vi"("error in (no error)"=w285, "VI Server Cluster"=w283) -> ("error out"=w284:errorcluster)  [unwired: 9 in]
          }
          event "Ch2.ReceivedDataArray.Index": Value Change {
            w288 = TRUE ("SingleInstance")
            n86 = event-data() -> ()  [unwired: 1 in, 2 out]
            n87 = call-poly "VI Server_GetControl_Value_Ref.vi"("DataType"=dbl[] [], "Control.Label"="Ch2.ReceivedDataArray", "error in"=w301, "SingleInstance"=w288, "VI Server.RefsCluster"=w300) -> ("error out"=w297:errorcluster, "Value"=w294:dbl[], "VI Server.RefsCluster.DUP"=w296:T5)  [unwired: 3 in, 1 out]
            n88 = call-poly "VI Server_GetControl_Value_Ref.vi"("DataType"=0, "Control.Label"="Ch2.ReceivedDataArray.Index", "error in"=w297, "SingleInstance"=w288, "VI Server.RefsCluster"=w296) -> ("error out"=w289:errorcluster, "Value"=w292:i32, "VI Server.RefsCluster.DUP"=w291:T5)  [unwired: 3 in, 1 out]
            n89 = Index Array(array=w294, index=w292) -> (element=w290:dbl)
            n90 = call-poly "VI Server_SetControl.vi"("Data"=w290, "Control.Label"="Ch2.ReceivedDataArray.IndexedValue", "error in"=w289, "SingleInstance"=w288, "VI Server.RefsCluster"=w291) -> ("error out"=w286:errorcluster)  [unwired: 4 in, 2 out]
          }
        }
        n91 = event shown="[1] \"CH1.TX.Frames.Cluster\", \"CH1.TX.Frame.Selector\", \"CH1.TX.Frame.Signals\", \"CH1.RX.Frames.Cluster\", \"CH1.RX.Frame.Selector\", \"CH1.RX.Frame.Signals\", \"CH1.TX.Signal.Data\": Value Change" {
          selector: _ -> [_ _ _ _ _ _ _ _ _ _ _ _ _ _ _ _ _ _ _ _ _ _]
          dyn-events: _ -> [_ _ _ _ _ _ _ _ _ _ _ _ _ _ _ _ _ _ _ _ _ _]
          timeout: 250 -> [_ _ _ _ _ _ _ _ _ _ _ _ _ _ _ _ _ _ _ _ _ _]
          tunnel: w29 -> [w40 w41 w50 w58 w64 w70 w76 w82 w88 w95 w102 w106 w110 w113 w116 w119 w122 w125 w128 w131 w135 w141]
          tunnel: [w40 w42 w51 w56 w62 w68 w75 w81 w87 w94 w101 w105 w107 w111 w114 w117 w120 w123 w127 w130 w134 w140] -> w26
          tunnel: w30 -> [_ w43 w52 w57 w63 w69 w74 w80 w89 w96 w103 w104 w108 w112 w115 w118 w121 w124 _ _ _ _]
          event Timeout {
            n92 = event-data() -> ()  [unwired: 1 in, 1 out]
          }
          event "CH1.TX.Frames.Cluster", "CH1.TX.Frame.Selector", "CH1.TX.Frame.Signals", "CH1.RX.Frames.Cluster", "CH1.RX.Frame.Selector", "CH1.RX.Frame.Signals", "CH1.TX.Signal.Data": Value Change {
            n93 = event-data() -> ("CtlRef"=w44:refnum<vi>)  [unwired: 1 in]
            n94 = To More Generic Class(target class=refnum<vi> refnum ("Control Reference (Generic)"), reference=w44) -> (generic class reference=w46:refnum<vi>)
            n95 = call "VECTOR 1610_Register_User_Last_Action.vi"("CtlRef"=w46, "error in (no error)"=w41, "VI Server Cluster"=w43) -> ("error out"=w42:errorcluster)  [unwired: 7 in, 1 out]
          }
          event "Ch1.TX.Transmit.Byte1", "Ch1.TX.Transmit.Byte2", "Ch1.TX.Transmit.Byte3", "Ch1.TX.Transmit.Byte4", "Ch1.TX.Transmit.Byte5", "Ch1.TX.Transmit.Byte6", "Ch1.TX.Transmit.Byte7", "Ch1.TX.Transmit.Byte8": Value Change {
            n96 = event-data() -> ("CtlRef"=w48:refnum<vi>)  [unwired: 1 in]
            n97 = To More Generic Class(target class=refnum<vi> refnum ("Control Reference (Generic)"), reference=w48) -> (generic class reference=w47:refnum<vi>)
            n98 = call "VECTOR 1610_Register_User_Last_Action.vi"("CtlRef"=w47, "error in (no error)"=w50, "VI Server Cluster"=w52) -> ("error out"=w51:errorcluster)  [unwired: 7 in, 1 out]
          }
          event "Ch1.TX.Payload": Value Change {
            n99 = event-data() -> ("CtlRef"=w55:refnum<vi>)  [unwired: 1 in]
            n100 = To More Generic Class(target class=refnum<vi> refnum ("Control Reference (Generic)"), reference=w55) -> (generic class reference=w53:refnum<vi>)
            n101 = call "VECTOR 1610_Register_User_Last_Action.vi"("CtlRef"=w53, "error in (no error)"=w58, "VI Server Cluster"=w57) -> ("error out"=w56:errorcluster)  [unwired: 7 in, 1 out]
          }
          event "CH1.TX.FrameID": Value Change {
            n102 = event-data() -> ("CtlRef"=w60:refnum<vi>)  [unwired: 1 in]
            n103 = To More Generic Class(target class=refnum<vi> refnum ("Control Reference (Generic)"), reference=w60) -> (generic class reference=w59:refnum<vi>)
            n104 = call "VECTOR 1610_Register_User_Last_Action.vi"("CtlRef"=w59, "error in (no error)"=w64, "VI Server Cluster"=w63) -> ("error out"=w62:errorcluster)  [unwired: 7 in, 1 out]
          }
          event "CH1.RX.FrameIDs": Value Change {
            n105 = event-data() -> ("CtlRef"=w66:refnum<vi>)  [unwired: 1 in]
            n106 = To More Generic Class(target class=refnum<vi> refnum ("Control Reference (Generic)"), reference=w66) -> (generic class reference=w65:refnum<vi>)
            n107 = call "VECTOR 1610_Register_User_Last_Action.vi"("CtlRef"=w65, "error in (no error)"=w70, "VI Server Cluster"=w69) -> ("error out"=w68:errorcluster)  [unwired: 7 in, 1 out]
          }
          event "Ch1.TX.DataLength": Value Change {
            n108 = event-data() -> ("CtlRef"=w72:refnum<vi>)  [unwired: 1 in]
            n109 = To More Generic Class(target class=refnum<vi> refnum ("Control Reference (Generic)"), reference=w72) -> (generic class reference=w71:refnum<vi>)
            n110 = call "VECTOR 1610_Register_User_Last_Action.vi"("CtlRef"=w71, "error in (no error)"=w76, "VI Server Cluster"=w74) -> ("error out"=w75:errorcluster)  [unwired: 7 in, 1 out]
          }
          event "Ch1.TX.Transmit", "Ch1.TX.Payload.Clear": Value Change {
            n111 = event-data() -> ("CtlRef"=w78:refnum<vi>)  [unwired: 1 in]
            n112 = To More Generic Class(target class=refnum<vi> refnum ("Control Reference (Generic)"), reference=w78) -> (generic class reference=w77:refnum<vi>)
            n113 = call "VECTOR 1610_Register_User_Last_Action.vi"("CtlRef"=w77, "error in (no error)"=w82, "VI Server Cluster"=w80) -> ("error out"=w81:errorcluster)  [unwired: 7 in, 1 out]
          }
          event "CH1.TX.Frames.Cluster", "CH1.RX.Frames.Cluster", "CH1.RX.Frame.Selector", "CH1.RX.Frame.Signals", "CH1.TX.Frame.Selector", "CH1.TX.Frame.Signals": Shortcut Menu Selection (User) {
            n114 = event-data() -> ("CtlRef"=w84:refnum<vi>, "ItemTag"=w86:string)  [unwired: 1 in]
            n115 = To More Generic Class(target class=refnum<vi> refnum ("Control Reference (Generic)"), reference=w84) -> (generic class reference=w83:refnum<vi>)
            n116 = call "VECTOR 1610_Controls_UserMenu.vi"("ItemTag"=w86, "Control Ref"=w83, "error in (no error)"=w88, "VI Server Cluster"=w89) -> ("error out"=w87:errorcluster)  [unwired: 7 in]
          }
          event "Ch1.TX.Transmit.Byte1", "Ch1.TX.Transmit.Byte2", "Ch1.TX.Transmit.Byte3", "Ch1.TX.Transmit.Byte4", "Ch1.TX.Transmit.Byte5", "Ch1.TX.Transmit.Byte6", "Ch1.TX.Transmit.Byte7", "Ch1.TX.Transmit.Byte8": Shortcut Menu Selection (User) {
            n117 = event-data() -> ("CtlRef"=w91:refnum<vi>, "ItemTag"=w93:string)  [unwired: 1 in]
            n118 = To More Generic Class(target class=refnum<vi> refnum ("Control Reference (Generic)"), reference=w91) -> (generic class reference=w90:refnum<vi>)
            n119 = call "VECTOR 1610_Controls_UserMenu.vi"("ItemTag"=w93, "Control Ref"=w90, "error in (no error)"=w95, "VI Server Cluster"=w96) -> ("error out"=w94:errorcluster)  [unwired: 7 in]
          }
          event "Ch1.TX.Payload", "CH1.TX.FrameID", "Ch1.TX.DataLength", "Ch1.TX.Transmit", "Ch1.TX.Payload.Clear", "CH1.RX.FrameIDs", "CH1.TX.Signal.Data": Shortcut Menu Selection (User) {
            n120 = event-data() -> ("CtlRef"=w98:refnum<vi>, "ItemTag"=w100:string)  [unwired: 1 in]
            n121 = To More Generic Class(target class=refnum<vi> refnum ("Control Reference (Generic)"), reference=w98) -> (generic class reference=w97:refnum<vi>)
            n122 = call "VECTOR 1610_Controls_UserMenu.vi"("ItemTag"=w100, "Control Ref"=w97, "error in (no error)"=w102, "VI Server Cluster"=w103) -> ("error out"=w101:errorcluster)  [unwired: 7 in]
          }
          event "LastAction.AddToSecuence": Value Change {
            n123 = event-data() -> ()  [unwired: 1 in, 1 out]
            n124 = call "VECTOR 1610_UserLastAction_Add_To_Sequence.vi"("error in (no error)"=w106, "VI Server Cluster"=w104) -> ("error out"=w105:errorcluster)  [unwired: 9 in]
          }
          event "TestCaseConfiguration": Shortcut Menu Selection (User) {
            n125 = event-data() -> ("ItemTag"=w109:string)  [unwired: 1 in]
            n126 = call "VECTOR1610_Sequence_TestCaseConfig_UserMenu.vi"("ItemTag"=w109, "error in (no error)"=w110, "VI Server.RefsCluster"=w108) -> ("error out"=w107:errorcluster)  [unwired: 8 in]
          }
          event "TestCaseConfiguration": Value Change {
            n127 = event-data() -> ()  [unwired: 1 in, 1 out]
            n128 = call "VECTOR 1610_TestCase_Configuration_ValueChanged.vi"("error in"=w113, "VI Server.RefsCluster"=w112) -> ("error out"=w111:errorcluster)  [unwired: 8 in, 1 out]
          }
          event "TestCase.SAVE": Value Change {
            n129 = event-data() -> ()  [unwired: 1 in, 1 out]
            n130 = call "VECTOR 1610_Sequence_Save.vi"("error in (no error)"=w116, "VI Server Cluster"=w115) -> ("error out"=w114:errorcluster)  [unwired: 9 in]
          }
          event "SequenceFile.Open": Value Change {
            n131 = event-data() -> ()  [unwired: 1 in, 1 out]
            n132 = call "VECTOR 1610_Sequence_Open.vi"("error in (no error)"=w119, "VI Server Cluster"=w118) -> ("error out"=w117:errorcluster)  [unwired: 9 in]
          }
          event "TestCase.Execute.All": Value Change {
            n133 = event-data() -> ()  [unwired: 1 in, 1 out]
            n134 = call "VECTOR 1610_Execute_All_Instruction.vi"("error in (no error)"=w122, "VI Server Cluster"=w121) -> ("error out"=w120:errorcluster)  [unwired: 9 in]
          }
          event "TestCase.Execute.Selected": Value Change {
            n135 = event-data() -> ()  [unwired: 1 in, 1 out]
            n136 = call "VECTOR 1610_ExecuteSelectedInstruction.vi"("error in (no error)"=w125, "VI Server Cluster"=w124) -> ("error out"=w123:errorcluster)  [unwired: 9 in]
          }
          event "TestCase.Execute.Pause": Value Change {
            n137 = event-data() -> ("NewVal"=w126:bool)  [unwired: 1 in]
            n138 = call "VECTOR1610_Accessor_Sequence_Execution_Pause_Ref.vi"() -> ("SequenceExecution.PAUSE"=w129:refnum<notifier>)  [unwired: 6 in]
            n139 = Send Notification(notification=w126, notifier=w129, error in (no error)=w128) -> (error out=w127:errorcluster)  [unwired: 1 out]
          }
          event "TestCase.Execute.Next": Value Change {
            n140 = event-data() -> ()  [unwired: 1 in, 1 out]
            n141 = call "VECTOR1610_Accessor_Sequence_Execution_NEXT_Ref.vi"() -> ("SequenceExecution.NEXT"=w133:refnum<notifier>)  [unwired: 6 in]
            n142 = Send Notification(notification=TRUE, notifier=w133, error in (no error)=w131) -> (error out=w130:errorcluster)  [unwired: 1 out]
          }
          event "TestCase.Execute.ABORT": Value Change {
            n143 = event-data() -> ()  [unwired: 1 in, 1 out]
            n144 = call "VECTOR1610_Accessor_Sequence_Execution_ABORT_Ref.vi"() -> ("SequenceExecution.ABORT"=w136:refnum<notifier>)  [unwired: 6 in]
            n145 = Send Notification(notification=TRUE, notifier=w136, error in (no error)=w135) -> (error out=w134:errorcluster)  [unwired: 1 out]
          }
          event "TestCase.Execute.Step.Pause": Value Change {
            n146 = event-data() -> ("NewVal"=w139:bool)  [unwired: 1 in]
            n147 = call "VECTOR1610_TestCase_Execution_Pause_Ref.vi"() -> ("SequenceExecution.StepPAUSE"=w138:refnum<notifier>)  [unwired: 6 in]
            n148 = Send Notification(notification=w139, notifier=w138, error in (no error)=w141) -> (error out=w140:errorcluster)  [unwired: 1 out]
          }
        }
        n149 = call "VECTOR 1610_Accessor_EXIT_Ref.vi"() -> ("EXIT"=w32:refnum<notifier>)  [unwired: 6 in]
        n150 = call "StopOnErrorOrCommand.vi"("STOP"=w32, "error in (no error)"=w34) -> ("error out"=w28:errorcluster, "STOP"=w33:bool)  [unwired: 8 in]
        n151 = call "Merge Errors II.vi"("error in 2 (no error)"=w26, "error in 1 (no error)"=w28) -> ("error out.DUP"=w27:errorcluster)  [unwired: 4 in, 1 out]
      }
      n152 = call "VECTOR 1610_UDP_MAIN.vi"("error in (no error)"=w18, "VI Server.RefsCluster"=w19) -> ("error out"=w24:errorcluster)  [unwired: 9 in]
      n153 = call "VECTOR 1610_CAN INTERFACE MAIN.vi"("error in (no error)"=w18, "VI Server Cluster"=w19) -> ("error out"=w20:errorcluster)  [unwired: 9 in]
      n154 = call "VECTORE 1610_Execute_Instructions_Processor.vi"("error in (no error)"=w18, "VI Server.RefsCluster"=w19) -> ("error out"=w17:errorcluster)  [unwired: 9 in]
      n155 = Build Array(w17, w20, w24) -> (w21:errorcluster[])
      n156 = call "Merge Errors II.vi"("error array in"=w21, "error in 1 (no error)"=w23) -> ("error out.DUP"=w22:errorcluster)  [unwired: 4 in, 1 out]
    }
    frame Error {
    }
  }
  n157 = call "VI Server_CloseRefs.vi"("error in"=w3, "VI Server.RefsCluster"=w4) -> ("error out"=w7:errorcluster)  [unwired: 9 in]
  n158 = call "VECTOR 1610_Synch_CLOSE.vi"("error in"=w7) -> ("error out"=w2:errorcluster)  [unwired: 10 in]
  n159 = Current VI's Path() -> (path=w6:path)
  n160 = call <vilib>:"Simple Error Handler.vi"("error in (no error)"=w2) -> ()  [unwired: 4 in, 5 out]
  n161 = call "Close Window If in EXE mode.vi"("TopLevelVI Path"=w6, "error in"=w2) -> ("error out"=→"error out":errorcluster)  [unwired: 9 in]
